vi "Reinitialize Default Values.vi"(8 "error in (no error)":errorcluster, 11 "VI in":refnum<vi>) -> (0 "error out":errorcluster)   [LabVIEW 2019]
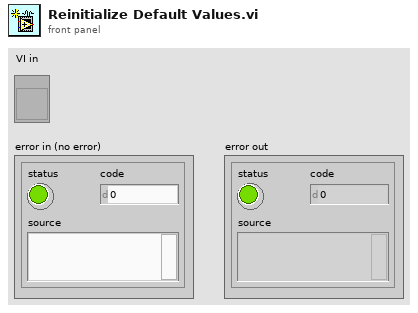
[diagram p1: front panel]
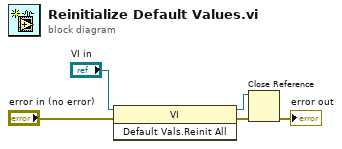
[diagram p0: block diagram]
diagram:
  n1 = invoke class="VI" method="Default Vals.Reinit All"(reference="VI in", error in="error in (no error)") -> (reference out=w3:refnum<vi>, error out=w2:errorcluster)  [unwired: 1 in, 1 out]
  n2 = Close Reference(reference=w3, error in (no error)=w2) -> (error out=→"error out":errorcluster)
